vi "TSM SSC Digital Log HRAM Results.vi"(0 "Digital TSM In":T3, 1 "Pattern Name":string, 2 "Destination Dir":path, 5 "Per-Site Cycle Information":T1[][](array[typedef]) {"actual pin states" items=["0"=0, "1"=1, "L"=3, "H"=4, "X"=5, "M"=6, "V"=7, "D"=8, "E"=9, "Not A Pin State"=254, "Pin State Not Acquired"=255]; "expected pin states" items=["0"=0, "1"=1, "L"=3, "H"=4, "X"=5, "M"=6, "V"=7, "D"=8, "E"=9, "Not A Pin State"=254, "Pin State Not Acquired"=255]}, 7 "Per-Site Scan Cycle Numbers":i64[][](array[numeric]) format="%.0x", 11 "error in":errorcluster) -> (4 "Digital TSM Out":T3, 6 "Files Generated":path[](array[path]), 15 "error out":errorcluster)   [LabVIEW 2019]
doc: "Fetches a defined number of samples for the sites connected to the specified pin(s) and pin group(s). This VI only returns data from sites that are enabled when fetch is called. Returns an array of per-site per-sample data where rows correspond to sites and columns correspond to samples."
uses:
  TSM/TSM SSC Digital.ctl
  <vilib>/NI_TestStand_SemiconductorModule/NI_TestStand_Semiconductor_Module.lvlibp/PinMap/Digital Pattern/PinQueryContext/DigitalPatternPinQueryContext.lvclass
  SSC Digital/SSC Digital.ctl
  <instrlib>/niDigital/niDigital.llb/niDigital History RAM Cycle Information (1D Pin States).ctl
  <instrlib>/niDigital/niDigital.llb/niDigital Pin State.ctl
  <vilib>/Utility/file.llb/Write Delimited Spreadsheet (string).vi
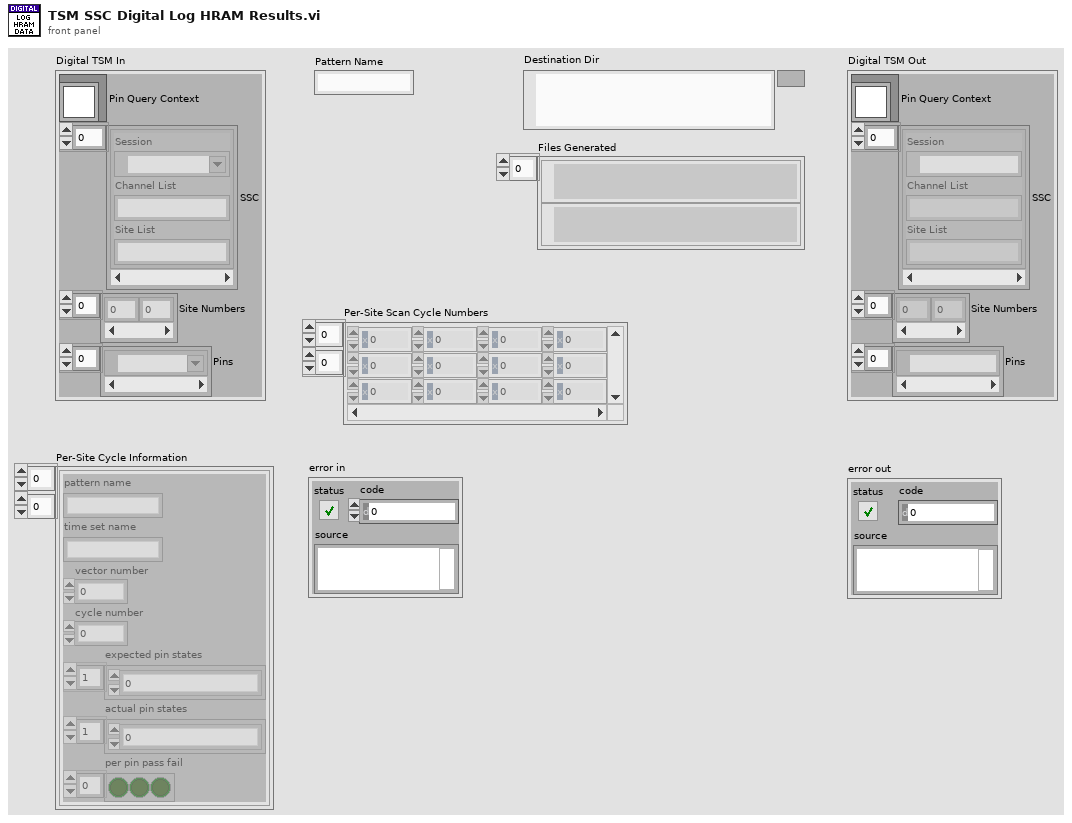
[diagram p1: front panel]
types:
  T1 = typedef "niDigital History RAM Cycle Information (1D Pin States).ctl" = cluster{"pattern name":string, "time set name":string, "vector number":i64, "cycle number":i64, "expected pin states":T2[], "actual pin states":T2[], "per pin pass fail":bool[]}
  T2 = typedef "niDigital Pin State.ctl" = u8
  T3 = typedef "TSM SSC Digital.ctl" = cluster{"Pin Query Context":refnum<class "DigitalPatternPinQueryContext.lvclass">, "SSC":T4[], "Site Numbers":i32[], "Pins":tag[]}
  T4 = typedef "SSC Digital.ctl" = cluster{"Session":refnum<k15>, "Channel List":string, "Site List":string}
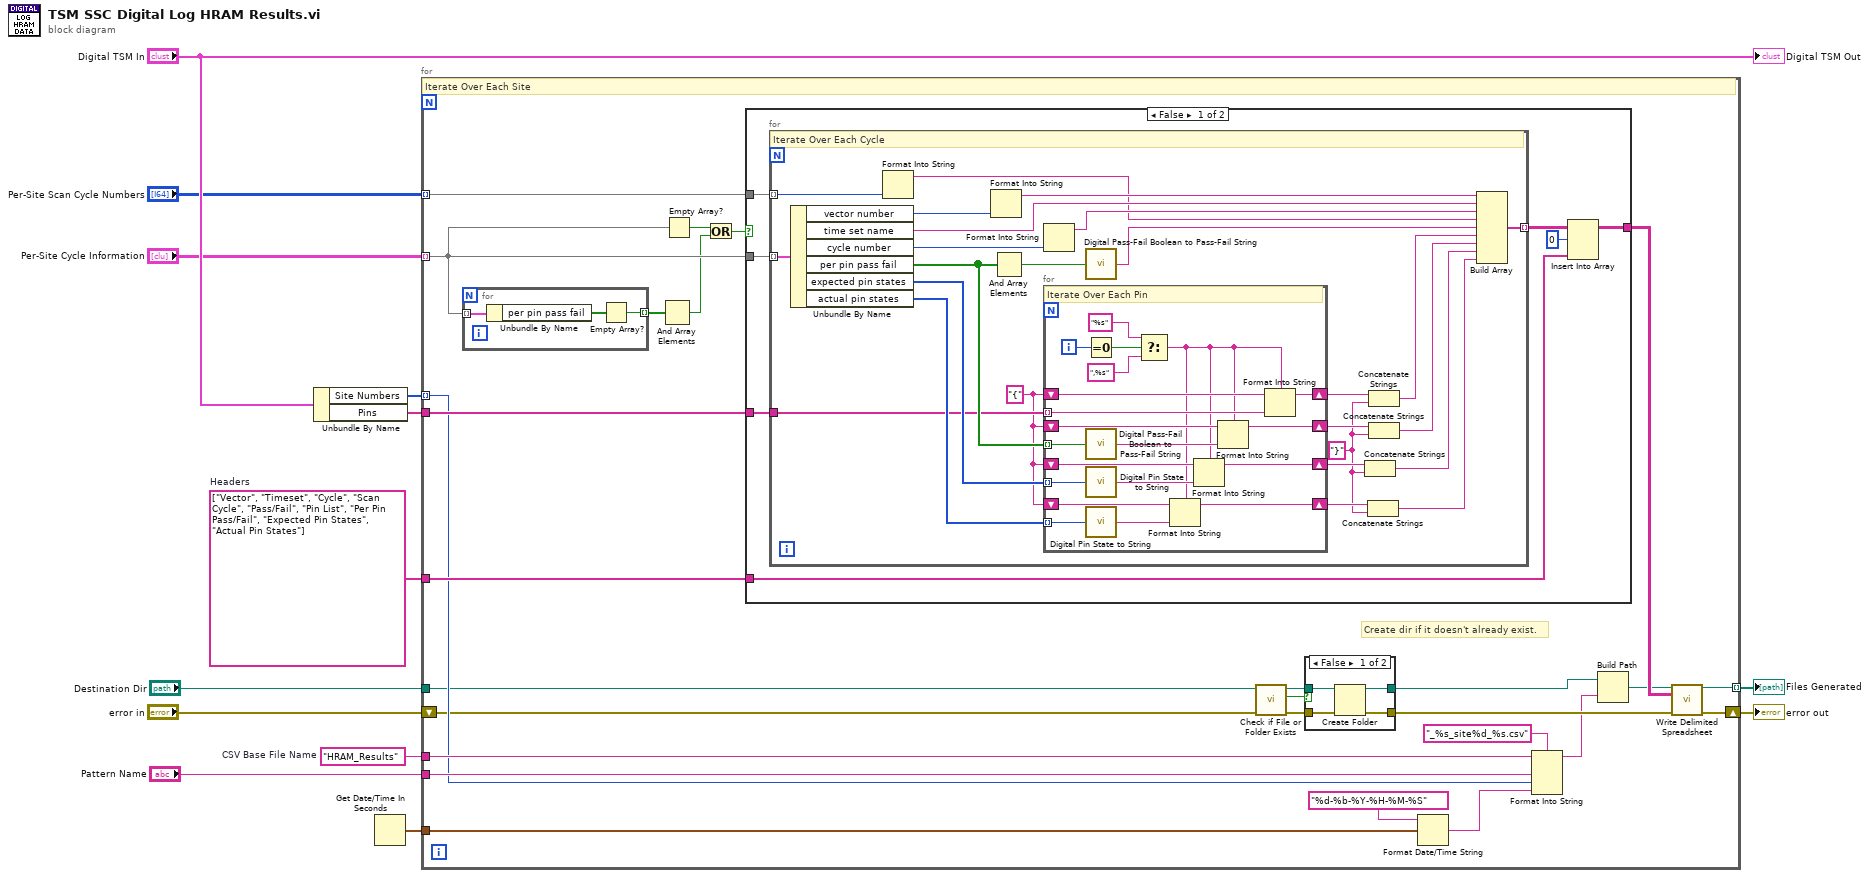
[diagram p0: block diagram]
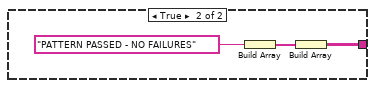
[diagram p3: hidden frame]
diagram:
  w6 = string[] ["Vector", "Timeset", "Cycle", "Scan Cycle", "Pass/Fail", "Pin List", "Per Pin Pass/Fail", "Expected Pin States", "Actual Pin States"]  # Headers
  w10 = "HRAM_Results"  # CSV Base File Name
  n1 = Unbundle By Name("Digital TSM In") -> ("Site Numbers"=w9:i32[], "Pins"=w2:tag[])
  n2 = Get Date/Time In Seconds() -> (seconds since 1Jan1904=w5:timestamp)
  n3 = for {
    tunnel: "Destination Dir" -> [w21]
    shift-right: [w39] -> w12
    shift-left: "error in" -> [w22]
    tunnel: w10 -> [w38]
    tunnel: w9 -> [w33] mode=indexing
    tunnel: [w37] -> w8 mode=indexing
    tunnel: "Per-Site Cycle Information" -> [w18] mode=indexing
    tunnel: "Per-Site Scan Cycle Numbers" -> [w31] mode=indexing
    tunnel: w6 -> [w36]
    tunnel: w5 -> [w35]
    tunnel: "Pattern Name" -> [w34]
    tunnel: w2 -> [w40]
    # "Create dir if it doesn't already exist."
    # "Iterate Over Each Site"
    n4 = for {
      tunnel: w18 -> [w43] mode=indexing
      tunnel: [w41] -> w16 mode=indexing
      n5 = Unbundle By Name(w43) -> ("per pin pass fail"=w42:bool[])
      n6 = Empty Array?(array=w42) -> (empty?=w41:bool)
    }
    n7 = And Array Elements(Boolean array=w16) -> (logical AND=w15:bool)
    n8 = Empty Array?(array=w18) -> (empty?=w32:bool)
    n9 = Or(x=w32, y=w15) -> (x .or. y?=w17:bool)
    n10 = case shown="False" w17 {
      tunnel: w18 -> [w56 _]
      tunnel: w36 -> [w54 _]
      tunnel: [w52 w102] -> w30
      tunnel: w40 -> [w51 _]
      tunnel: w31 -> [w50 _]
      frame False {
        n11 = for {
          tunnel: w56 -> [w78] mode=indexing
          tunnel: [w74] -> w55 mode=indexing
          tunnel: w51 -> [w60]
          tunnel: w50 -> [w57] mode=indexing
          w63 = "}" ("format string")
          w59 = "{" ("format string")
          # "Iterate Over Each Cycle"
          n12 = Unbundle By Name(w78) -> ("vector number"=w77:i64, "time set name"=w70:string, "cycle number"=w71:i64, "per pin pass fail"=w69:bool[], "expected pin states"=w68:T2[], "actual pin states"=w67:T2[])
          n13 = Format Into String(w57) -> (resulting string=w58:string)  [unwired: 3 in, 1 out]
          n14 = Format Into String(w77) -> (resulting string=w73:string)  [unwired: 3 in, 1 out]
          n15 = And Array Elements(Boolean array=w69) -> (logical AND=w76:bool)
          n16 = Format Into String(w71) -> (resulting string=w72:string)  [unwired: 3 in, 1 out]
          n17 = for {
            shift-right: [w98] -> w81
            shift-left: w59 -> [w99]
            shift-right: [w93] -> w80
            shift-left: w59 -> [w92]
            shift-right: [w91] -> w79
            shift-left: w59 -> [w90]
            tunnel: w69 -> [w86] mode=indexing
            tunnel: w68 -> [w85] mode=indexing
            tunnel: w67 -> [w84] mode=indexing
            shift-right: [w83] -> w61
            shift-left: w59 -> [w100]
            tunnel: w60 -> [w101] mode=indexing
            i -> [w97]
            # "Iterate Over Each Pin"
            n18 = Equal To 0?(x=w97) -> (x = 0?=w95:bool)
            n19 = call "Digital Pass-Fail Boolean to Pass-Fail String.vi"("Pass/Fail"=w86) -> ("Pass/Fail String"=w89:string)  [unwired: 14 in]
            n20 = call "Digital Pin State to String.vi"("Pin State"=w85) -> ("String"=w88:string)  [unwired: 14 in]
            n21 = call "Digital Pin State to String.vi"("Pin State"=w84) -> ("String"=w87:string)  [unwired: 14 in]
            n22 = Select(t="%s" ("format string"), s=w95, f=",%s") -> (s? t:f=w82:string)
            n23 = Format Into String(format string=w82, initial string=w90, w87) -> (resulting string=w91:string)  [unwired: 1 in, 1 out]
            n24 = Format Into String(format string=w82, initial string=w92, w88) -> (resulting string=w93:string)  [unwired: 1 in, 1 out]
            n25 = Format Into String(format string=w82, initial string=w99, w89) -> (resulting string=w98:string)  [unwired: 1 in, 1 out]
            n26 = Format Into String(format string=w82, initial string=w100, w101) -> (resulting string=w83:string)  [unwired: 1 in, 1 out]
          }
          n27 = call "Digital Pass-Fail Boolean to Pass-Fail String.vi"("Pass/Fail"=w76) -> ("Pass/Fail String"=w75:string)  [unwired: 14 in]
          n28 = Concatenate Strings(w80, w63) -> (w66:string)
          n29 = Concatenate Strings(w79, w63) -> (w65:string)
          n30 = Concatenate Strings(w61, w63) -> (w62:string)
          n31 = Concatenate Strings(w81, w63) -> (w64:string)
          n32 = Build Array(w73, w70, w72, w58, w75, w62, w64, w66, w65) -> (w74:string[])
        }
        n33 = Insert Into Array(array=w55, index (row)=0, new element=w54) -> (w52:string[][])  [unwired: 1 in]
      }
      frame True {
        n34 = Build Array("PATTERN PASSED - NO FAILURES" ("String")) -> (w103:string[])
        n35 = Build Array(w103) -> (w102:string[][])
      }
    }
    n36 = call <vilib>:"Check if File or Folder Exists.vi"("error in (no error)"=w22, "path"=w21) -> ("error out"=w25:errorcluster, "file or folder exists?"=w23:bool, "dup path"=w24:path)  [unwired: 7 in]
    n37 = case shown="False" w23 {
      tunnel: w25 -> [w47 w49]
      tunnel: w24 -> [w46 w48]
      tunnel: [w45 w48] -> w19
      tunnel: [w44 w49] -> w20
      frame False {
        n38 = Create Folder(path (use dialog)=w46, error in=w47) -> (created path=w45:path, error out=w44:errorcluster)  [unwired: 1 in, 1 out]
      }
      frame True {
      }
    }
    n39 = Format Date/Time String(time format string (%c)="%d-%b-%Y-%H-%M-%S", seconds (now)=w35) -> (date/time string=w28:string)  [unwired: 1 in]
    n40 = Format Into String(format string="_%s_site%d_%s.csv", initial string=w38, w34, w33, w28) -> (resulting string=w14:string)  [unwired: 1 in, 1 out]
    n41 = Build Path(base path=w19, name or relative path=w14) -> (appended path=w29:path)
    n42 = call-poly <vilib>:"Write Delimited Spreadsheet.vi"("file path (dialog if empty)"=w29, "2D data"=w30, "error in (no error)"=w20) -> ("new file path (Not A Path if cancelled)"=w37:path, "error out"=w39:errorcluster)  [unwired: 11 in]
  }
  "error out" <- w12
  "Files Generated" <- w8
  "Digital TSM Out" <- "Digital TSM In"
